vi "Display_ScanNextPixel.vi"() -> (15 "ActivePixel":T2, 18 "ActiveTile":T1)   [LabVIEW 2018]
uses:
  TypDefs/ActivePixel_Cluster.ctl
  TypDefs/ActiveTile_Cluster.ctl
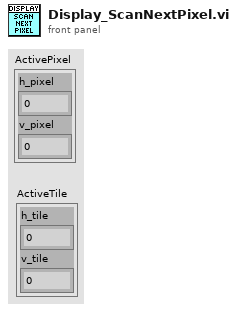
[diagram p1: front panel]
types:
  T1 = typedef "ActiveTile_Cluster.ctl" = cluster{"h_tile":i16, "v_tile":i16}
  T2 = typedef "ActivePixel_Cluster.ctl" = cluster{"h_pixel":i16, "v_pixel":i16}
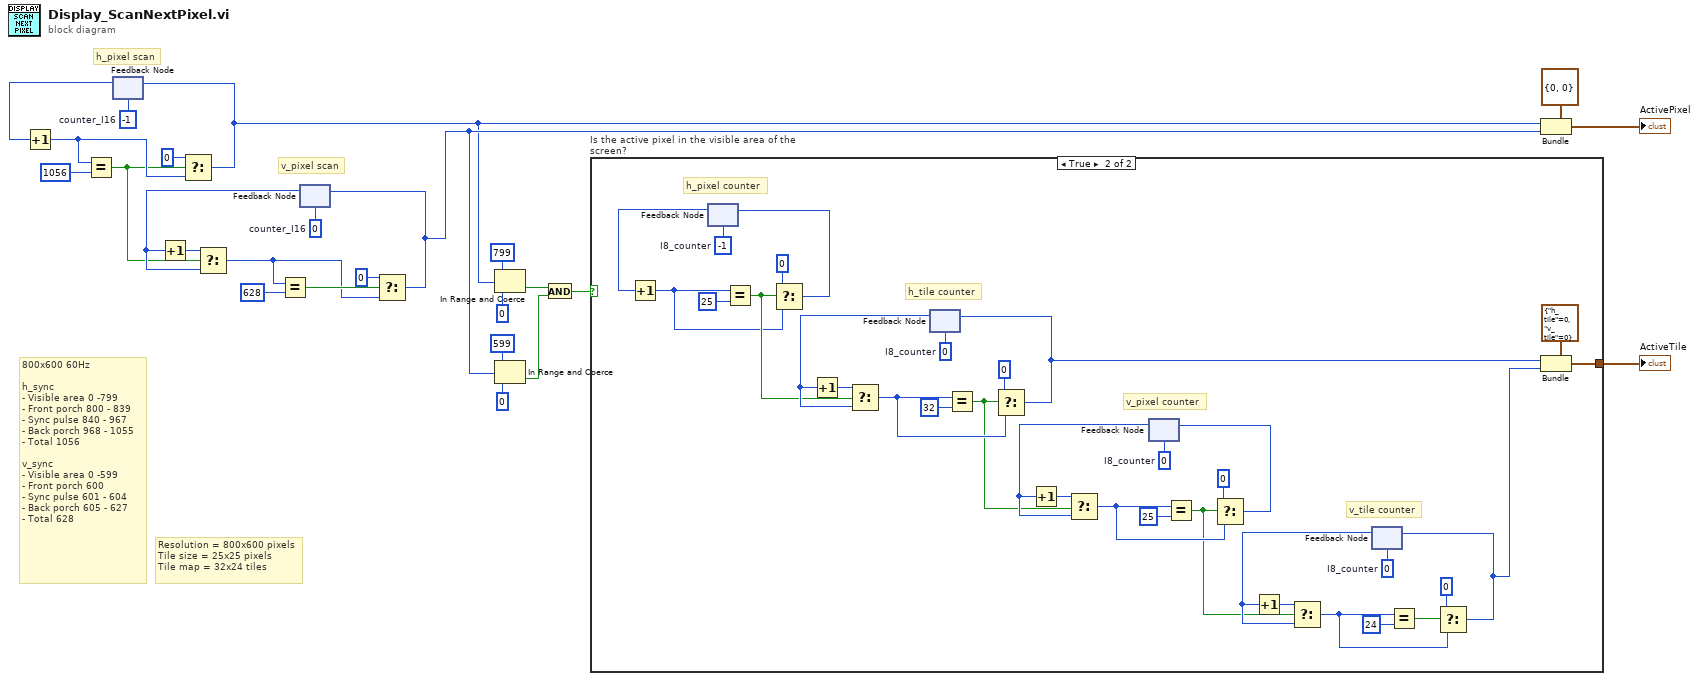
[diagram p0: block diagram]
diagram:
  w18 = i16 0  # counter_I16
  w22 = i16 -1  # counter_I16
  # "Resolution = 800x600 pixels\nTile size = 25x25 pixels\nTile map = 32x24 tiles"
  # "v_pixel scan"
  # "h_pixel scan"
  # "800x600 60Hz\n\nh_sync\n- Visible area 0 -799\n- Front porch 800 - 839\n- Sync pulse 840 - 967\n- Back porch 968 - 1055\n- Total 1056\n\nv_sync\n- Visible area 0 -599\n- Front porch 600\n- Sync pulse 601 - 604\n- Back porch 605 - 627\n- Total 628"
  n1 = feedback #1(w22) -> (w21:i16)
  n2 = Increment(x=w21) -> (x+1=w24:i16)
  n3 = Equal?(x=w24, y=i16 1056) -> (x = y?=w12:bool)
  n4 = Select(t=i16 0 ("f"), s=w12, f=w24) -> (s? t:f=w2:i16)
  n5 = feedback-in #1(w2) -> ()
  n6 = feedback #2(w18) -> (w14:i16)
  n7 = Increment(x=w14) -> (x+1=w16:i16)
  n8 = Select(t=w16, s=w12, f=w14) -> (s? t:f=w15:i16)
  n9 = Equal?(x=w15, y=i16 628) -> (x = y?=w17:bool)
  n10 = Select(t=i16 0 ("f"), s=w17, f=w15) -> (s? t:f=w3:i16)
  n11 = feedback-in #2(w3) -> ()
  n12 = In Range and Coerce(upper limit=i16 799, x=w2, lower limit=i16 0) -> (In Range?=w7:bool)  [unwired: 1 out]
  n13 = In Range and Coerce(upper limit=i16 599, x=w3, lower limit=i16 0) -> (In Range?=w4:bool)  [unwired: 1 out]
  n14 = And(x=w7, y=w4) -> (x .and. y?=w1:bool)
  n15 = case "Is the active pixel in the visible area of the screen?" shown="True" w1 {
    tunnel: [_ w58] -> w10
    frame False {
    }
    frame True {
      w32 = i8 -1  # I8_counter
      w40 = i8 0  # I8_counter
      w48 = i8 0  # I8_counter
      w55 = i8 0  # I8_counter
      # "h_pixel counter"
      # "v_tile counter"
      # "v_pixel counter"
      # "h_tile counter"
      n16 = feedback #3(w32) -> (w33:i8)
      n17 = Increment(x=w33) -> (x+1=w26:i8)
      n18 = Equal?(x=w26, y=i8 25) -> (x = y?=w29:bool)
      n19 = Select(t=i8 0, s=w29, f=w26) -> (s? t:f=w34:i8)
      n20 = feedback-in #3(w34) -> ()
      n21 = feedback #4(w55) -> (w53:i8)
      n22 = Increment(x=w53) -> (x+1=w54:i8)
      n23 = Select(t=w54, s=w29, f=w53) -> (s? t:f=w52:i8)
      n24 = Equal?(x=w52, y=i8 32) -> (x = y?=w28:bool)
      n25 = Select(t=i8 0, s=w28, f=w52) -> (s? t:f=w45:i8)
      n26 = feedback-in #4(w45) -> ()
      n27 = feedback #5(w48) -> (w50:i8)
      n28 = Increment(x=w50) -> (x+1=w49:i8)
      n29 = Select(t=w49, s=w28, f=w50) -> (s? t:f=w51:i8)
      n30 = Equal?(x=w51, y=i8 25) -> (x = y?=w27:bool)
      n31 = Select(t=i8 0, s=w27, f=w51) -> (s? t:f=w44:i8)
      n32 = feedback-in #5(w44) -> ()
      n33 = feedback #6(w40) -> (w38:i8)
      n34 = Increment(x=w38) -> (x+1=w39:i8)
      n35 = Select(t=w39, s=w27, f=w38) -> (s? t:f=w37:i8)
      n36 = Equal?(x=w37, y=i8 24) -> (x = y?=w43:bool)
      n37 = Select(t=i8 0, s=w43, f=w37) -> (s? t:f=w36:i8)
      n38 = feedback-in #6(w36) -> ()
      n39 = Bundle(cluster=T1 {"h_tile"=0, "v_tile"=0} ("position"), "h_tile"=w45, "v_tile"=w36) -> (w58:T1)
    }
  }
  "ActiveTile" <- w10
  n40 = Bundle(cluster=T2 {"h_pixel"=0, "v_pixel"=0} ("position"), "h_pixel"=w2, "v_pixel"=w3) -> (→"ActivePixel":T2)
